vi "ma_manage_buffer.vi"(7 "Initialize":bool, 10 "Y":dbl[](array[numeric]) format="%0.2f", 11 "state info":T1 {"buffer" format="%0.2f"; "timestamp" format="%<%.4X>T"; "dt history" format="%0.2f"; "t0 history" format="%<%I:%M:%S%4u %p>T"; "exp TC (samples)" format="%0.2f"; "RMS history" format="%0.2f"; "DC history" format="%0.2f"}) -> (1 "#blocks":i32, 2 "Output Array":dbl[][](array[numeric]) format="%0.2f", 3 "state info":T1 {"buffer" format="%0.2f"; "timestamp" format="%<%.4X>T"; "dt history" format="%0.2f"; "t0 history" format="%<%I:%M:%S%4u %p>T"; "exp TC (samples)" format="%0.2f"; "RMS history" format="%0.2f"; "DC history" format="%0.2f"})   [LabVIEW 2020, in "NI_MAPro.lvlib"]
uses:
  NI_MAPro.lvlib
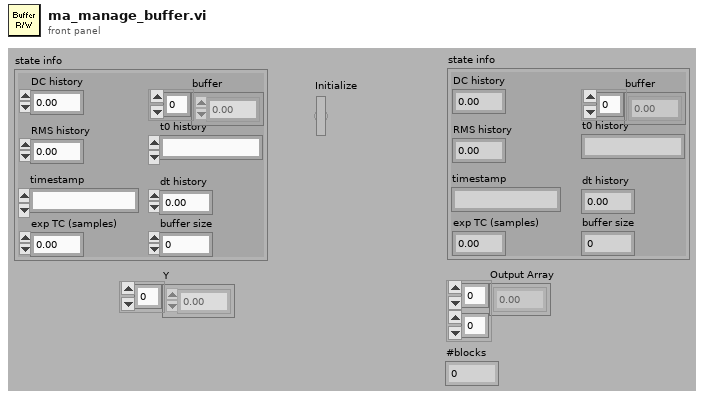
[diagram p1: front panel]
types:
  T1 = cluster{"DC history":dbl, "RMS history":dbl, "exp TC (samples)":dbl, "buffer size":i32, "t0 history":timestamp, "dt history":dbl, "timestamp":timestamp, "buffer":dbl[]}
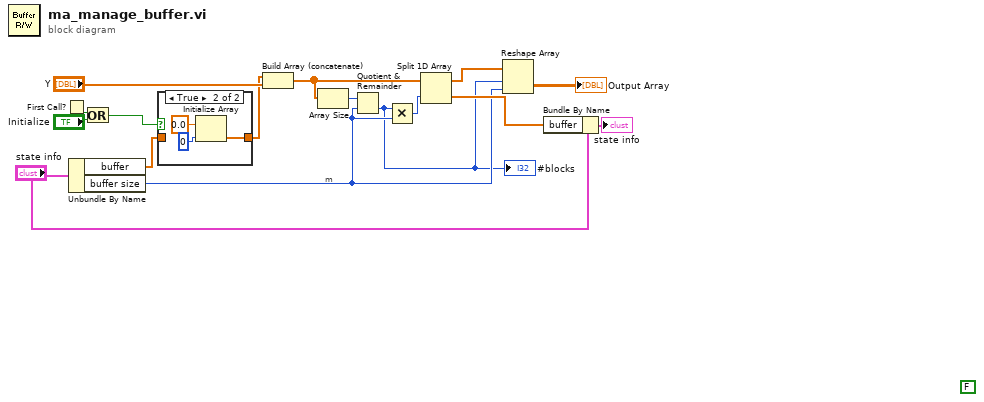
[diagram p0: block diagram]
diagram:
  (unwired) FALSE
  # "m"
  n1 = First Call?() -> (First Call?: T/F=w15:bool)
  n2 = Unbundle By Name("state info") -> ("buffer"=w7:dbl[], "buffer size"=w3:i32)
  n3 = Or(x=w15, y="Initialize") -> (x .or. y?=w1:bool)
  n4 = case shown="True" w1 {
    tunnel: [w17 w20] -> w9
    tunnel: w7 -> [w17 _]
    frame False {
    }
    frame True {
      n5 = Initialize Array(0.0 ("Element Data"), 0 ("Dimension Size")) -> (w20:dbl[])
    }
  }
  n6 = Build Array (concatenate)(w9, "Y") -> (w11:dbl[])
  n7 = Array Size(array=w11) -> (size(s)=w12:i32)
  n8 = Quotient & Remainder(x=w12, y=w3) -> (floor(x/y)=w2:i32)  [unwired: 1 out]
  "#blocks" <- w2
  n9 = Multiply(x=w2, y=w3) -> (x*y=w10:i32)
  n10 = Split 1D Array(array=w11, index=w10) -> (first subarray=w8:dbl[], second subarray=w5:dbl[])
  n11 = Reshape Array(w8, w2, w3) -> (→"Output Array":dbl[][])
  n12 = Bundle By Name(cluster="state info", "buffer"=w5) -> (→"state info":T1)
